vi "Get Port.vi"(0 "Simulated in":refnum<class "Simulated.lvclass">, 5 "VISA resource name":refnum<visa-resource-name>, 9 "Puerto":u8, 11 "error in (no error)":errorcluster) -> (4 "Simulated out":refnum<class "Simulated.lvclass">, 6 "VISA resource name 2":refnum<visa-resource-name>, 8 "bool response":bool[](array[boolean]), 10 "Response":string, 15 "error out":errorcluster)   [LabVIEW 2020, in "Simulated.lvclass"]
uses:
  Simulated.lvclass
  Abstract/Serial Device/Serial Device.lvclass
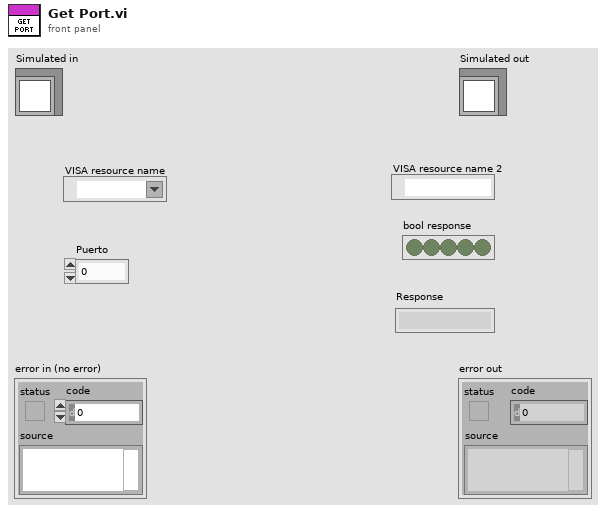
[diagram p1: front panel]
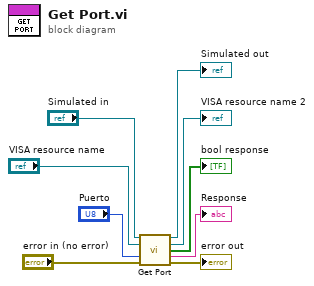
[diagram p0: block diagram]
diagram:
  n1 = call-parent "Get Port.vi"("Serial Device in"="Simulated in", "VISA resource name"="VISA resource name", "Puerto"="Puerto", "error in (no error)"="error in (no error)") -> ("Serial Device out"=→"Simulated out":refnum<class "Simulated.lvclass">, "VISA resource name 2"=→"VISA resource name 2":refnum<visa-resource-name>, "bool response"=→"bool response":bool[], "Response"=→"Response":string, "error out"=→"error out":errorcluster)  [unwired: 7 in]
